vi "SetMusicVolume.vi"(8 "error in (no error)":errorcluster, 10 "VolumeData":T1, 11 "Engine in":refnum<class "Engine.lvclass">) -> (0 "error out":errorcluster, 3 "Engine out":refnum<class "Engine.lvclass">)   [LabVIEW 2019, in "RT_Game.lvlib" / "Engine.lvclass"]
uses:
  Engine.lvclass
  ChangeVolumeData.ctl
  MessageCluster.ctl
  Engine.lvclass/Engine.ctl
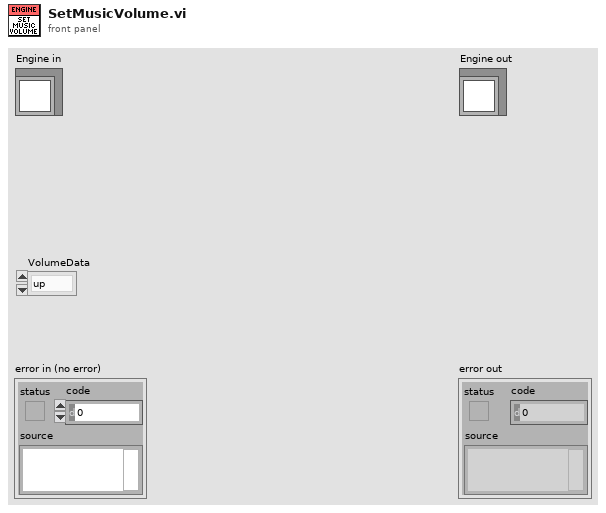
[diagram p1: front panel]
types:
  T1 = typedef "RT_Game.lvlib/Engine.lvclass/ChangeVolumeData.ctl" = enum16{"up", "down", "mute"}
  T2 = typedef "RT_Game.lvlib/Engine.lvclass/MessageCluster.ctl" = cluster{"Message":string, "Data":variant}
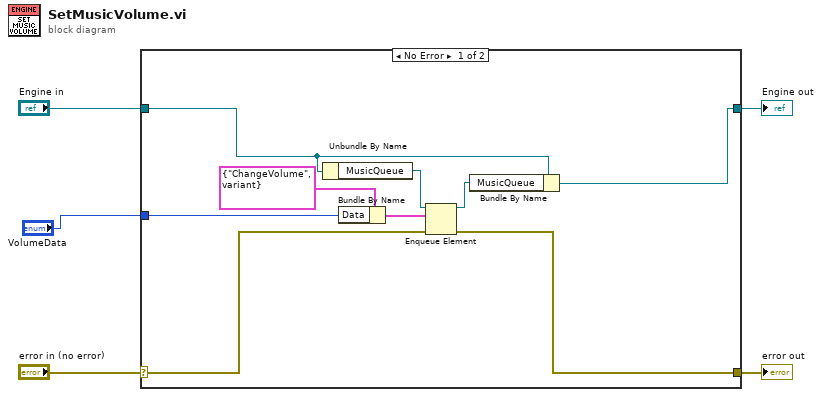
[diagram p0: block diagram]
diagram:
  n1 = case shown="No Error" "error in (no error)" {
    selector: "error in (no error)" -> [w7 w16]
    tunnel: [w8 w16] -> w4
    tunnel: [w9 w15] -> w2
    tunnel: "Engine in" -> [w10 w15]
    tunnel: "VolumeData" -> [w6 _]
    frame No Error {
      n2 = Unbundle By Name(w10) -> ("MusicQueue"=w11:refnum<queue>)
      n3 = Bundle By Name(cluster=T2 {"Message"="ChangeVolume", "Data"=variant} ("element"), "Data"=w6) -> (w14:T2)
      n4 = Enqueue Element(queue=w11, element=w14, error in (no error)=w7) -> (queue out=w12:refnum<queue>, error out=w8:errorcluster)  [unwired: 1 in, 1 out]
      n5 = Bundle By Name(cluster=w10, "MusicQueue"=w12) -> (w9:refnum<class "Engine.lvclass">)
    }
    frame Error {
    }
  }
  "error out" <- w4
  "Engine out" <- w2
